vi "ADC_Start.vi"(0 "GPIB Address":T1=8, 11 "error in (no error)":errorcluster) -> (15 "error out":errorcluster={"status"=FALSE, "code"=0, "source"="\nADC Start.vi"})   [LabVIEW 2010]
doc: "Triggers the ADC rack, if the ADC is configured to start from a GET.\nCould also start the BSA(s) if their addresses are included in the array"
uses:
  ADC_GPIB_address.ctl
panel:
  in  "?":bool
  # "GPIB GET"
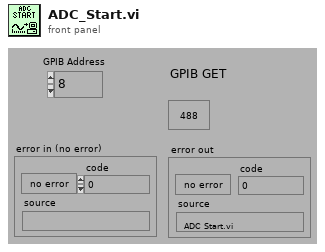
[diagram p1: front panel]
types:
  T1 = typedef "ADC_GPIB_address.ctl" = u8
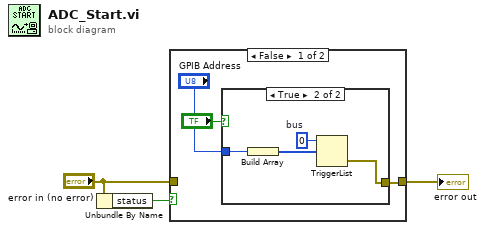
[diagram p0: block diagram]
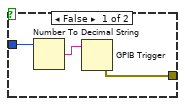
[diagram p2: hidden frame]
diagram:
  n1 = Unbundle By Name("error in (no error)") -> ("status"=w1:bool)
  n2 = case shown="False" w1 {
    tunnel: [w6 w14] -> w3
    tunnel: "error in (no error)" -> [_ w14]
    frame False {
      n3 = case shown="True" "?" {
        tunnel: "GPIB Address" -> [w9 w12]
        tunnel: [w7 w10] -> w6
        frame False {
          n4 = Number To Decimal String(number=w9) -> (decimal integer string=w8:string)  [unwired: 1 out]
          n5 = GPIB Trigger(3:w8) -> (0:w7:errorcluster)  [unwired: 1 in, 1 out]
        }
        frame True {
          w11 = 0  # bus
          n6 = Build Array(w12) -> (w13:T1[])
          n7 = TriggerList(3:w13, 4:w11) -> (0:w10:errorcluster)  [unwired: 1 in, 1 out]
        }
      }
    }
    frame True {
    }
  }
  "error out" <- w3
